vi "example_move.vi"   [LabVIEW 2023]
uses:
  Terminal/Terminal.lvclass
  C:/projects/TLC_Scripto/Source/GObject/GObject.lvclass
  BlockDiagram/Read controlTerminals.vi
  BlockDiagram/BlockDiagram.lvclass
  TLC_Scripto.lvlib
  GObject/GObject.lvclass
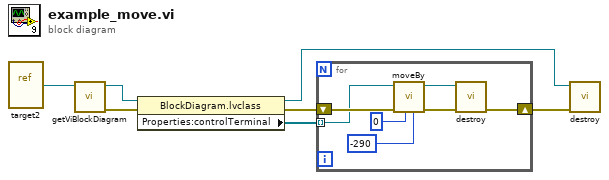
[diagram p0: block diagram]
diagram:
  n1 = vi-ref "target2.vi"() -> (w7:refnum<vi>)
  n2 = call "getViBlockDiagram.vi"("ViRef"=w7) -> ("error out"=w6:errorcluster, "topMostBlockDiagram"=w5:refnum<class "BlockDiagram.lvclass">)  [unwired: 9 in]
  n3 = property class="BlockDiagram.lvclass"(reference=w5, error in=w6) -> (reference out=w4:refnum<class "BlockDiagram.lvclass">, error out=w3:errorcluster, "Properties:controlTerminal"=w2:refnum<class "Terminal.lvclass">[])
  n4 = for {
    tunnel: w2 -> [w11] mode=indexing
    shift-right: [w10] -> w1
    shift-left: w3 -> [w14]
    n5 = call "moveBy.vi"("dy(vertical)"=-290, "dx(horiziontal)"=0, "error in (no error)"=w14, "GObject in"=w11) -> ("error out"=w12:errorcluster, "GObject out"=w13:refnum<class "Terminal.lvclass">)  [unwired: 6 in]
    n6 = call-dynamic "destroy.vi"("Error In"=w12, "Generic In"=w13) -> ("Error Out"=w10:errorcluster)  [unwired: 9 in]
  }
  n7 = call-dynamic "destroy.vi"("Error In"=w1, "Generic In"=w4) -> ()  [unwired: 9 in, 1 out]
